vi "VIPM Project Parser.vi"() -> ()   [LabVIEW 2019]
uses:
  Build/Project.Dependencies Finder.lvlibp/Dependency Source_VIPM/Dependency Source_VIPM.lvclass
  C:/Current projects/LV32.2019..ProjectDependenciesFinder/Build/Project.Dependencies Finder.lvlibp/Dependency Source/Dependency Source.lvclass
  Build/Project.Dependencies Finder.lvlibp/Dependency Source_NIPM/Dependency Source_NIPM.lvclass
  Build/Project.Dependencies Finder.lvlibp/Dependency Source_GPM/Dependency Source_GPM.lvclass
  Build/Project.Dependencies Finder.lvlibp
  Build/Project.Dependencies Finder.lvlibp/Ctl/Ctl_Internal Target Element.ctl
  Build/Project.Dependencies Finder.lvlibp/Ctl/Ctl_External Target Element.ctl
  GPM/gpm_packages/@cs/actor-framework-messages/Source/MessageCycle/Message Cycle Notifications.ctl
  GPM/gpm_packages/@cs/actor-framework-messages/Source/MessageCycle/MessageCycle.lvclass
panel:
  in  "Load Stored Targets?(T)":bool=TRUE
  out "Unhandled Targets":string[](array[string])
  out "External Dependencies":string[](array[string])
  out "Internal Dependencies":string[](array[string])
  out "Error Out":errorcluster
  in  "Project Path in":path=path "C:/Current projects/LV32.2019..ProjectDependenciesFinder/_Test/Test.lvproj"
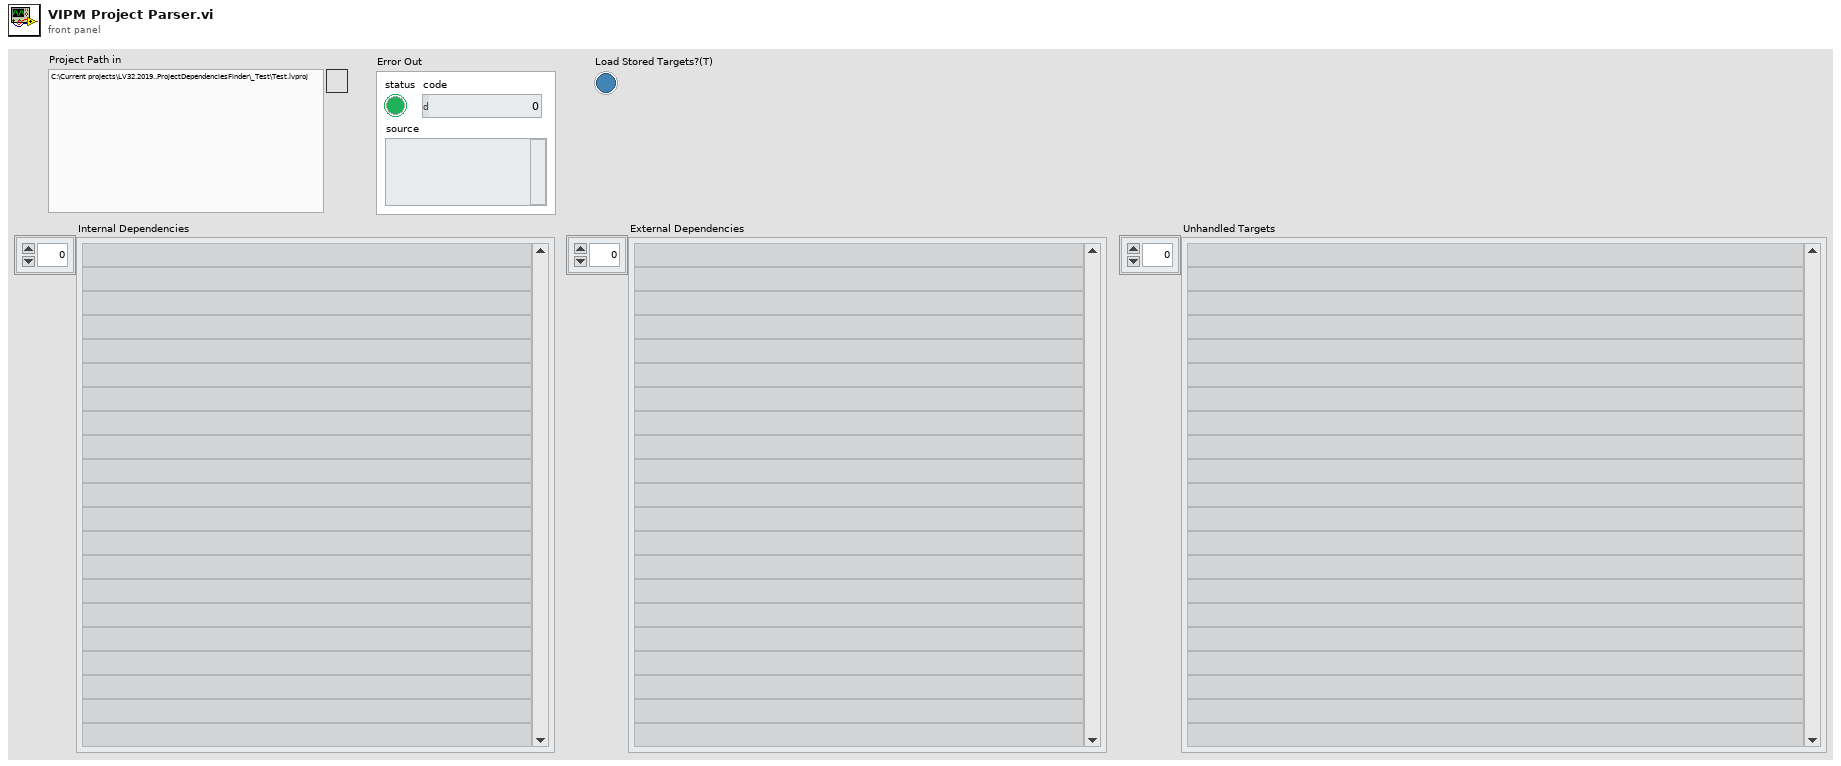
[diagram p1: front panel]
types:
  T1 = typedef "MessageCycle.lvclass/Message Cycle Notifications.ctl" = enum16{"Process Final Copy and Stop", "Stop Immediately", "Substitute Last Message and Stop"}
  T2 = typedef "Project.Dependencies Finder.lvlibp/Ctl_External Target Element.ctl" = cluster{"Target Source":string, "External Target Map":map{string, string}}
  T3 = typedef "Project.Dependencies Finder.lvlibp/Ctl_Internal Target Element.ctl" = cluster{"Target Source":string, "Internal Target Map":map{string, string}}
  T4 = typedef "Project.Dependencies Finder.lvlibp/Ctl_Dependency Element.ctl" = cluster{"Dependency Type":string, "Dependencies":string[]}
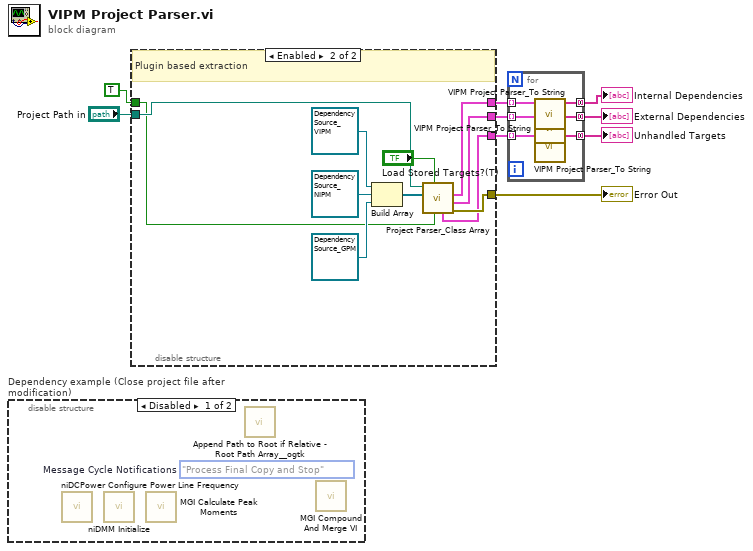
[diagram p0: block diagram]
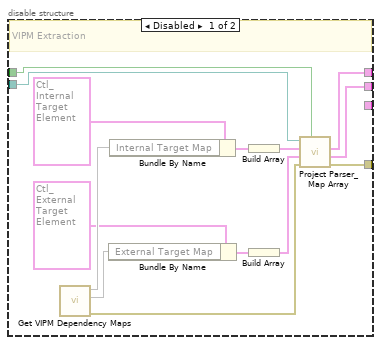
[diagram p2: hidden frame]
diagram:
  n1 = disable-structure "Dependency example (Close project file after modification)" shown="Disabled" {
    frame Disabled {
      (unwired) Message_Cycle_Notifications."Process Final Copy and Stop"  # Message Cycle Notifications
      n2 = call <instrlib>:"niDCPower Configure Power Line Frequency.vi"() -> ()  [unwired: 10 in, 2 out]
      n3 = call <instrlib>:"niDMM Initialize.vi"() -> ()  [unwired: 10 in, 2 out]
      n4 = call <userlib>:"MGI Calculate Peak Moments.vi"() -> ()  [unwired: 3 in, 3 out]
      n5 = call <userlib>:"Append Path to Root if Relative - Root Path Array__ogtk.vi"() -> ()  [unwired: 2 in, 1 out]
      n6 = call <userlib>:"MGI Compound And Merge VI.vi"() -> ()  [unwired: 1 in]
    }
    frame Enabled {
    }
  }
  n7 = disable-structure shown="Enabled" {
    disable-tunnel: "Project Path in" -> [w23 w34]
    disable-tunnel: [w22 w31] -> w8
    disable-tunnel: [w18 w33] -> w7
    disable-tunnel: [w17 w32] -> w4
    disable-tunnel: TRUE ("To Lower Case?(T)") -> [w16 w25]
    disable-tunnel: [_ w28] -> w2
    frame Disabled {
      # "VIPM Extraction"
      n8 = call "Get VIPM Dependency Maps.vi"() -> ("error out"=w10:errorcluster, "External Target Map"=w13:map{string, string}, "Internal Target Map"=w15:map{string, string})  [unwired: 7 in, 2 out]
      n9 = Bundle By Name(cluster=T2 {"Target Source"="VIPM", "External Target Map"={}} ("External Targets"), "External Target Map"=w13) -> (w12:T2)
      n10 = Bundle By Name(cluster=T3 {"Target Source"="VIPM", "Internal Target Map"={}} ("Internal Target Element"), "Internal Target Map"=w15) -> (w20:T3)
      n11 = Build Array(w20) -> (w19:T3[])
      n12 = Build Array(w12) -> (w11:T2[])
      n13 = call "Project Parser_Map Array.vi"("To Lower Case?(T)"=w16, "Error In"=w10, "External Targets"=w11, "Internal Targets"=w19, "Project Path in"=w23) -> ("Error Out"=w22:errorcluster, "Found External Dependencies"=w17:T4[], "Found Internal Dependencies"=w18:T4[])  [unwired: 3 in, 1 out]
    }
    frame Enabled {
      # "Plugin based extraction"
      n14 = Build Array(refnum<class "Dependency Source_VIPM.lvclass"> refnum ("Project.Dependencies Finder.lvlibp:Dependency Source_VIPM.lvclass"), refnum<class "Dependency Source_NIPM.lvclass"> refnum ("Project.Dependencies Finder.lvlibp:Dependency Source_NIPM.lvclass"), refnum<class "Dependency Source_GPM.lvclass"> refnum ("Project.Dependencies Finder.lvlibp:Dependency Source_GPM.lvclass")) -> (w29:refnum<class "Dependency Source.lvclass">[])
      n15 = call "Project Parser_Class Array.vi"("To Lower Case?(T)"=w25, "Load Stored Targets?(T)"="Load Stored Targets?(T)", "Dependency Source Plugins"=w29, "Project Path in"=w34) -> ("Error Out"=w31:errorcluster, "Found External Dependencies"=w32:T4[], "Found Internal Dependencies"=w33:T4[], "Unhandled Targets"=w28:T4[])  [unwired: 2 in, 2 out]
    }
  }
  "Error Out" <- w8
  n16 = for {
    tunnel: w7 -> [w37] mode=indexing
    tunnel: [w40] -> w6 mode=concatenating
    tunnel: [w39] -> w5 mode=concatenating
    tunnel: w4 -> [w35] mode=indexing
    tunnel: w2 -> [w36] mode=indexing
    tunnel: [w38] -> w1 mode=concatenating
    n17 = call "VIPM Project Parser_To String.vi"("External Target Element"=w37) -> ("Dependencies"=w40:string[])  [unwired: 10 in]
    n18 = call "VIPM Project Parser_To String.vi"("External Target Element"=w35) -> ("Dependencies"=w39:string[])  [unwired: 10 in]
    n19 = call "VIPM Project Parser_To String.vi"("External Target Element"=w36) -> ("Dependencies"=w38:string[])  [unwired: 10 in]
  }
  "Internal Dependencies" <- w6
  "External Dependencies" <- w5
  "Unhandled Targets" <- w1
